vi "GPS -Utility Show Locations.vi"() -> ()   [LabVIEW 2019]
uses:
  <vilib>/Utility/miscctls.llb/LVPoint32TypeDef.ctl
  SUBVIS/ctlGPSColIdxs.ctl
  SUBVIS/InputsGPSTool.ctl
  SUBVIS/ctlMode4GPSTool.ctl
  SUBVIS/ctlSeqFNs -GPSLocation.ctl
  SUBVIS/ctlGPSChangeMrksInputs.ctl
  SUBVIS/ctlInput4PtsColl.ctl
  System.Drawing
  SUBVIS/ctlAddrToGPSInputs.ctl
  C:/Users/WeGo/Documents/GitHub/ERP42mini-v2/GPS/gmap.net/GMAP.NET 8.6/data/GMap.NET.Core.dll
  data/GMap.NET.Core.dll
  SUBVIS/GLBL -GPSLocation.vi
  SUBVIS/GLOBAL -Project MAIN.vi
  C:/Users/WeGo/Documents/GitHub/ERP42mini-v2/GPS/gmap.net/GMAP.NET 8.6/data/GMap.NET.WindowsForms.dll
  data/GMap.NET.WindowsForms.dll
panel:
  in  "Inputs":T1={"ctlMode4GPSTool"=enum."Audit", "Addr"="Talisman Center", "City"="Calgary", "Prov"="Alberta", "Idx"=0, "Lat"="", "Lng"="", "Audited"=FALSE}
  in  "cmbProviders":string(combo)="27" caption="Map Providers"
  in  "tbCtl":enum32{"Audit"}(tab)
  in  "btnCancel":bool
  in  "btnUseMarkerShown":bool
  in  "Refersh":bool
  in  "ClearMarkers":bool
  in  "tbCtlGUI":enum32{"Position", "Pin Drop", "Addr", "Setup"}(tab)
  out "MouseLatDblClck":dbl caption="Lat" format="%#.7f"
  out "MouseLngDblClck":dbl caption="Lng" format="%#.7f"
  out "MouseLat":dbl caption="Lat" format="%#.7f"
  out "MouseLng":dbl caption="Lng" format="%#.7f"
  in  "GetNearPtsDyn":bool
  in  "# Pts":i32=5
  in  "GetNearPts":bool
  in  "PinDropMrkr":T3(ring) caption="Pin Drop Marker"
  out "PinDropLngDblClck":dbl caption="Lng:" format="%#.7f"
  out "PinDropLatDblClck":dbl caption="Lat:" format="%#.7f"
  out "AddrLng":dbl format="%#.7f"
  out "AddrLat":dbl format="%#.7f"
  in  "Get Lat+Lng":bool
  in  "City":string
  in  "Prov":string
  in  "Addr":string="20 Citadel Hills Green NW" caption="Address (Street level)"
  out "InitLoc":string="Calgary, Alberta" caption="Location Start KeyWords"
  out "InitProviders":string="GoogleMap" caption="Starting Provider"
  in  "Mode":T4(ring)
  in  "btnZoom+Center":bool
  in  "SaveImage":bool
  out "ImgPath":string caption="Path"
  in  "Zoom":dbl(slide) scale=0.0..20.0
  in  "tbctlHide":enum32{"Page 1", "Page 2"}(tab)
  out "error out":errorcluster
  in  "error in (no error)":errorcluster
  out "Coords":T5
  in  "EnumMarkerTypes":T3(ring)
  in  "ColIdxs":T6
  in  "Postion":T7
  in  "dotNetGMap":refnum<k24>(container)
  # "ABOVE is Marker LAT, LNG for ADRESS SHOWN:\n\n- If Marker Position is NOT Accurate:\n\n                           (1) 'Clear' the shown marker by clicking on <Clear Markers>\n\n                           (2) 'Double-Click' on Map to drop a Pin at New Position\n\n- If Marker Position is Accurate:\n                           \n                              Click Use the 'Marker Position' Shown to accept you new position"
  # "DYNAMIC"
  # "Mouse <Move> Coordinates"
  # "STATIC"
  # "Mouse <Dbl Clck> Coordinates"
  # "STEP 1. Dbl Clck Position"
  # "STEP 2. Edit Marker"
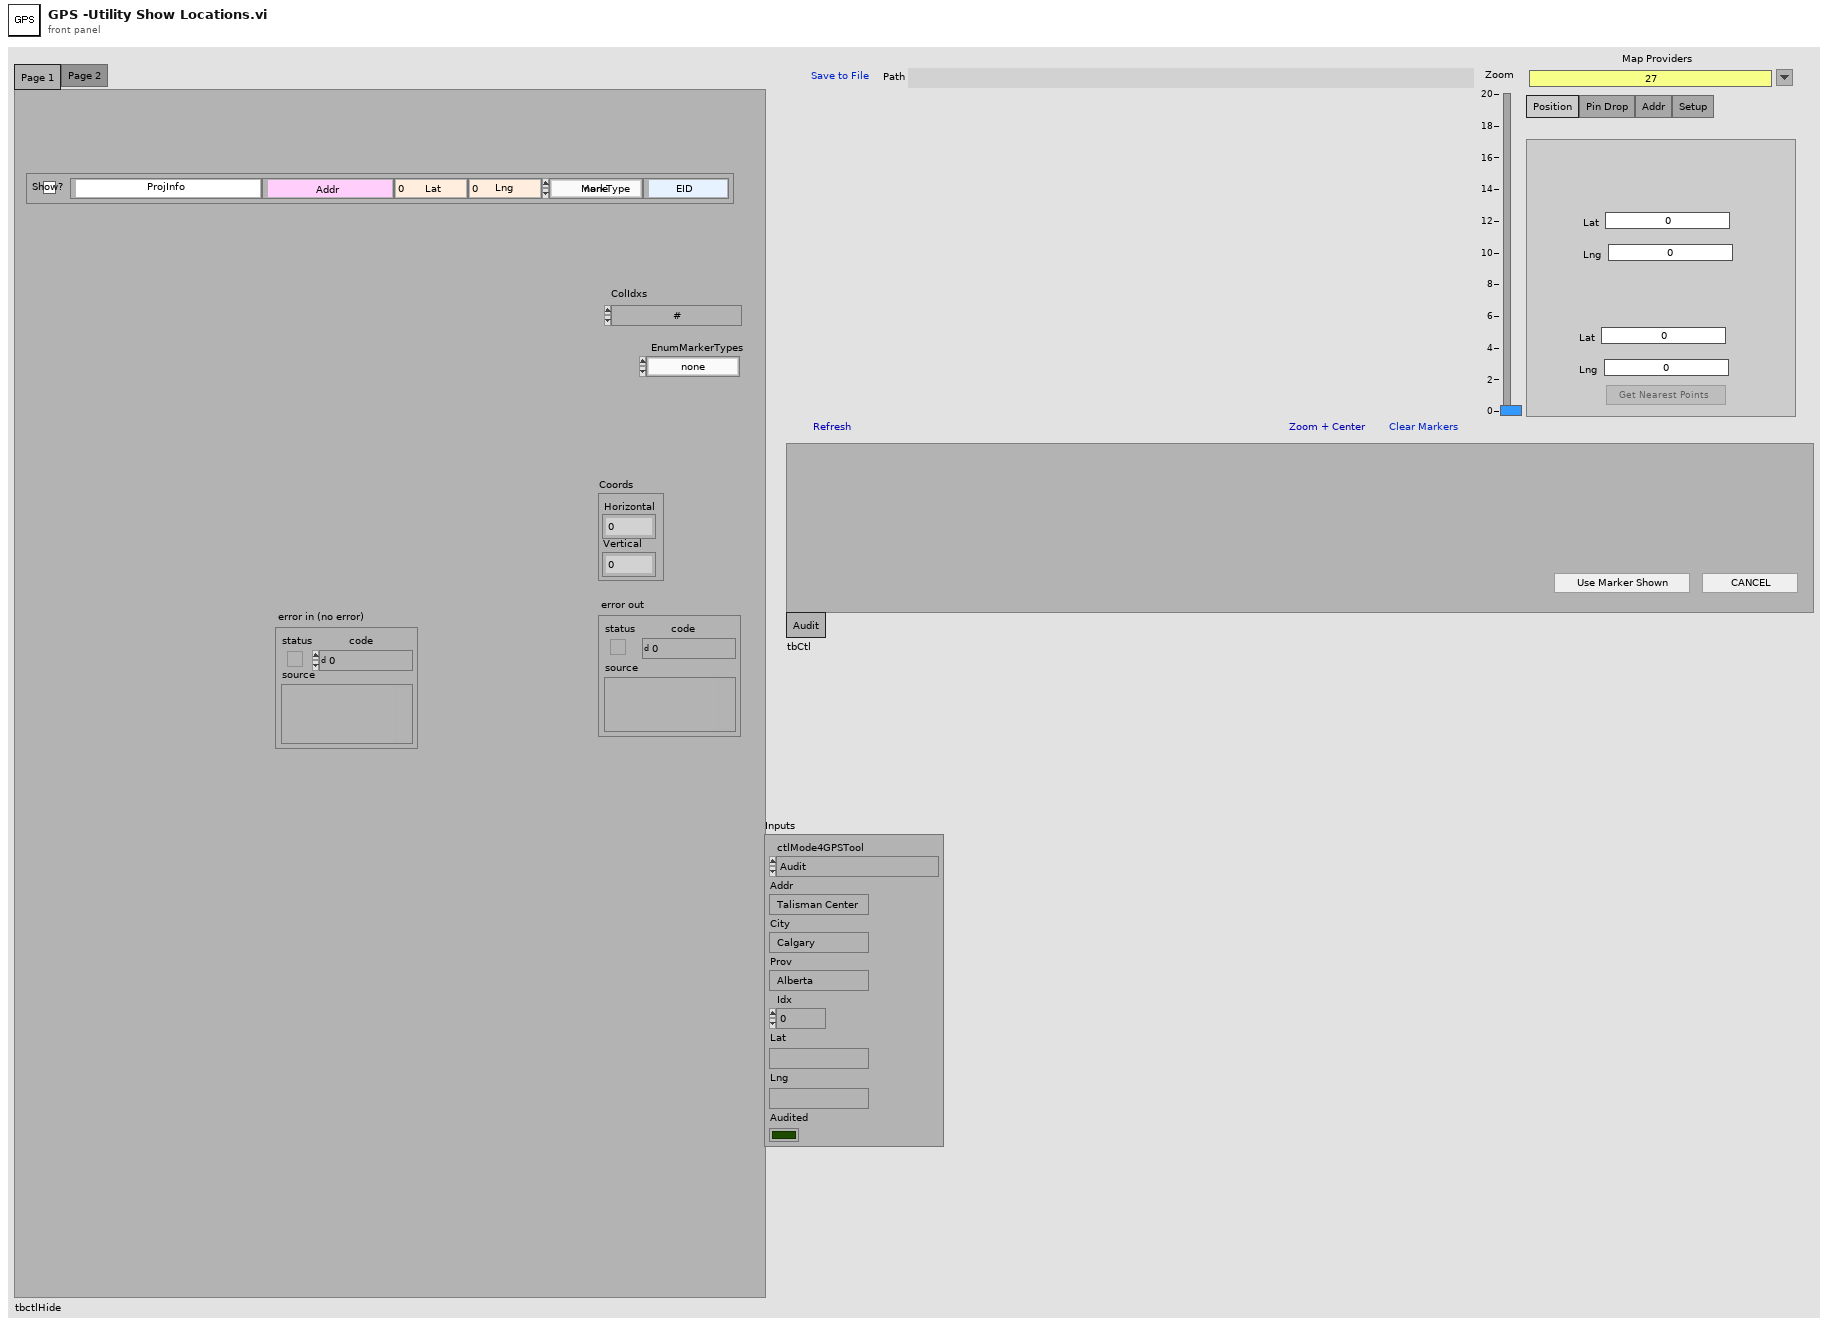
[diagram p1: front panel]
types:
  T1 = typedef "InputsGPSTool.ctl" = cluster{"ctlMode4GPSTool":T2, "Addr":string, "City":string, "Prov":string, "Idx":i32, "Lat":string, "Lng":string, "Audited":bool}
  T2 = typedef "ctlMode4GPSTool.ctl" = enum16{"NA", "Audit"}
  T3 = enum16{"none", "arrow", "blue", "blue_small", "blue_dot", "blue_pushpin", "brown_small", "gray_small", "green", "green_small", "green_dot", "green_pushpin", "green_big_go", "yellow", "yellow_small", "yellow_dot", "yellow_big_pause", "yellow_pushpin", "lightblue", "lightblue_dot", "lightblue_pushpin", "orange", "orange_small", "orange_dot", "pink", "pink_dot", "pink_pushpin", "purple", "purple_small", "purple_dot", "purple_pushpin", "red", "red_small", "red_dot", "red_pushpin", "red_big_stop", "black_small", "white_small"}
  T4 = enum16{"ServerOnly", "ServerAndCache", "CacheOnly"}
  T5 = typedef "LVPoint32TypeDef.ctl" = cluster{"Horizontal":i32, "Vertical":i32}
  T6 = typedef "ctlGPSColIdxs.ctl" = enum16{"#", "Vw", "Year", "Project Info", "Address", "Lat", "Lng", "Icon -Maps", "Icon -Custom", "EIDProj", "EIDAddr", "OnMap"}
  T7 = cluster{"Show?":bool, "ProjInfo":string, "Addr":string, "Lat":dbl, "Lng":dbl, "MarkType":enum16{"none", "arrow", "blue", "blue_small", "blue_dot", "blue_pushpin", "brown_small", "gray_small", "green", "green_small", "green_dot", "green_pushpin", "green_big_go", "yellow", "yellow_small", "yellow_dot", "yellow_big_pause", "yellow_pushpin", "lightblue", "lightblue_dot", "lightblue_pushpin", "orange", "orange_small", "orange_dot", "pink", "pink_dot", "pink_pushpin", "purple", "purple_small", "purple_dot", "purple_pushpin", "red", "red_small", "red_dot", "red_pushpin", "red_big_stop", "black_small", "white_small"}, "EID":string}
  T8 = typedef "ctlSeqFNs -GPSLocation.ctl" = enum16{"pre-init", "preinit01", "preinit02", "preinit03", "preinit04", "preinit05", "init", "idle", "GUI -Pop Menu", "GUI -Add Marker Combo", "GUI -Annotate Grid", "ALIGN COLS", "SET -Provider", "SET -SCALE", "OVERLAY -ADD", "POINTS -CREATE LIST (Container)", "MARKERS -CREATE LIST", "MAP -MARKER Add Or Rmv", "DOWNLOAD -Project Addr", "MAP -Marker Update", "MAP -Save", "MAP -Markers Autofit", "MAP -Addr to Lat + Lng", "MAP -Markers Clear", "PIN DROP -Get Nearest", "AUDIT -Use Marker Shown", "error", "exit"}
  T9 = cluster{"Idx|Addr|City|Prov|Lng|Lat|Checked":string[], "tbCtlGUI":refnum<vi>, "PinDropLatDblClck":refnum<vi>, "PinDropLngDblClck":refnum<vi>, "Cols4Show":i32, "ColHdrs":string[], "ColNos":i32[], "ColWidths":i32[], "AligmntEnum":i32[], "MouseLat":refnum<vi>, "MouseLng":refnum<vi>, "RefScale":refnum<vi>, "RefcmbProviders":refnum<vi>, "RefMode":refnum<vi>, "RefInitProvider":refnum<vi>, "EvntRefGMap":refnum<k27>, "arrRefProviders":refnum<k24>[], "arrProviderNms":string[], "RefInitLoc":refnum<vi>, "dotNetGMap":refnum<k24>, "PathCurr":path, "VIRef":refnum<vi>, "arrOverlayNames":string[], "arrOverlayRefs":refnum<k24>[], "RefPointsColl":refnum<k24>, "arrLatLngActv":dbl[][], "arrPointKeyWordOrID":string[], "EvntRefVsData":refnum<k27>, "MouseLatDblClck":refnum<vi>, "MouseLngDblClck":refnum<vi>, "Inputs":T1}
  T10 = enum8{"Enabled", "Disabled", "Disabled and Grayed Out"}
  T11 = typedef "ctlInput4PtsColl.ctl" = cluster{"arrLatLngActv":dbl[][], "ptKeyorID":string[], "Add":bool}
  T12 = cluster{"arrOverlayRefs":refnum<k24>[], "RefPointsColl in":refnum<k24>, "arrPointKeyWordOrID":string[], "PtLatLn+KywrdOrID":T11, "arrLatLngActv":dbl[][]}
  T13 = typedef "ctlAddrToGPSInputs.ctl" = cluster{"City":string, "State":string, "Addr":string, "EID":string}
  T14 = cluster{" # Pts":i32, "PinDropLatDblClck":dbl, "PinDropLngDblClck":dbl, "AddrLat":dbl, "AddrLng":dbl, "tbVw":enum32{"Position", "Pin Drop", "Addr", "Setup"}}
  T15 = cluster{refnum<vi>[], "tbCtlGUI":refnum<vi>, "queue out":refnum<queue>}
  T16 = typedef "ctlGPSChangeMrksInputs.ctl" = cluster{"r|c":i32[], "ID":string, "MrkName":string}
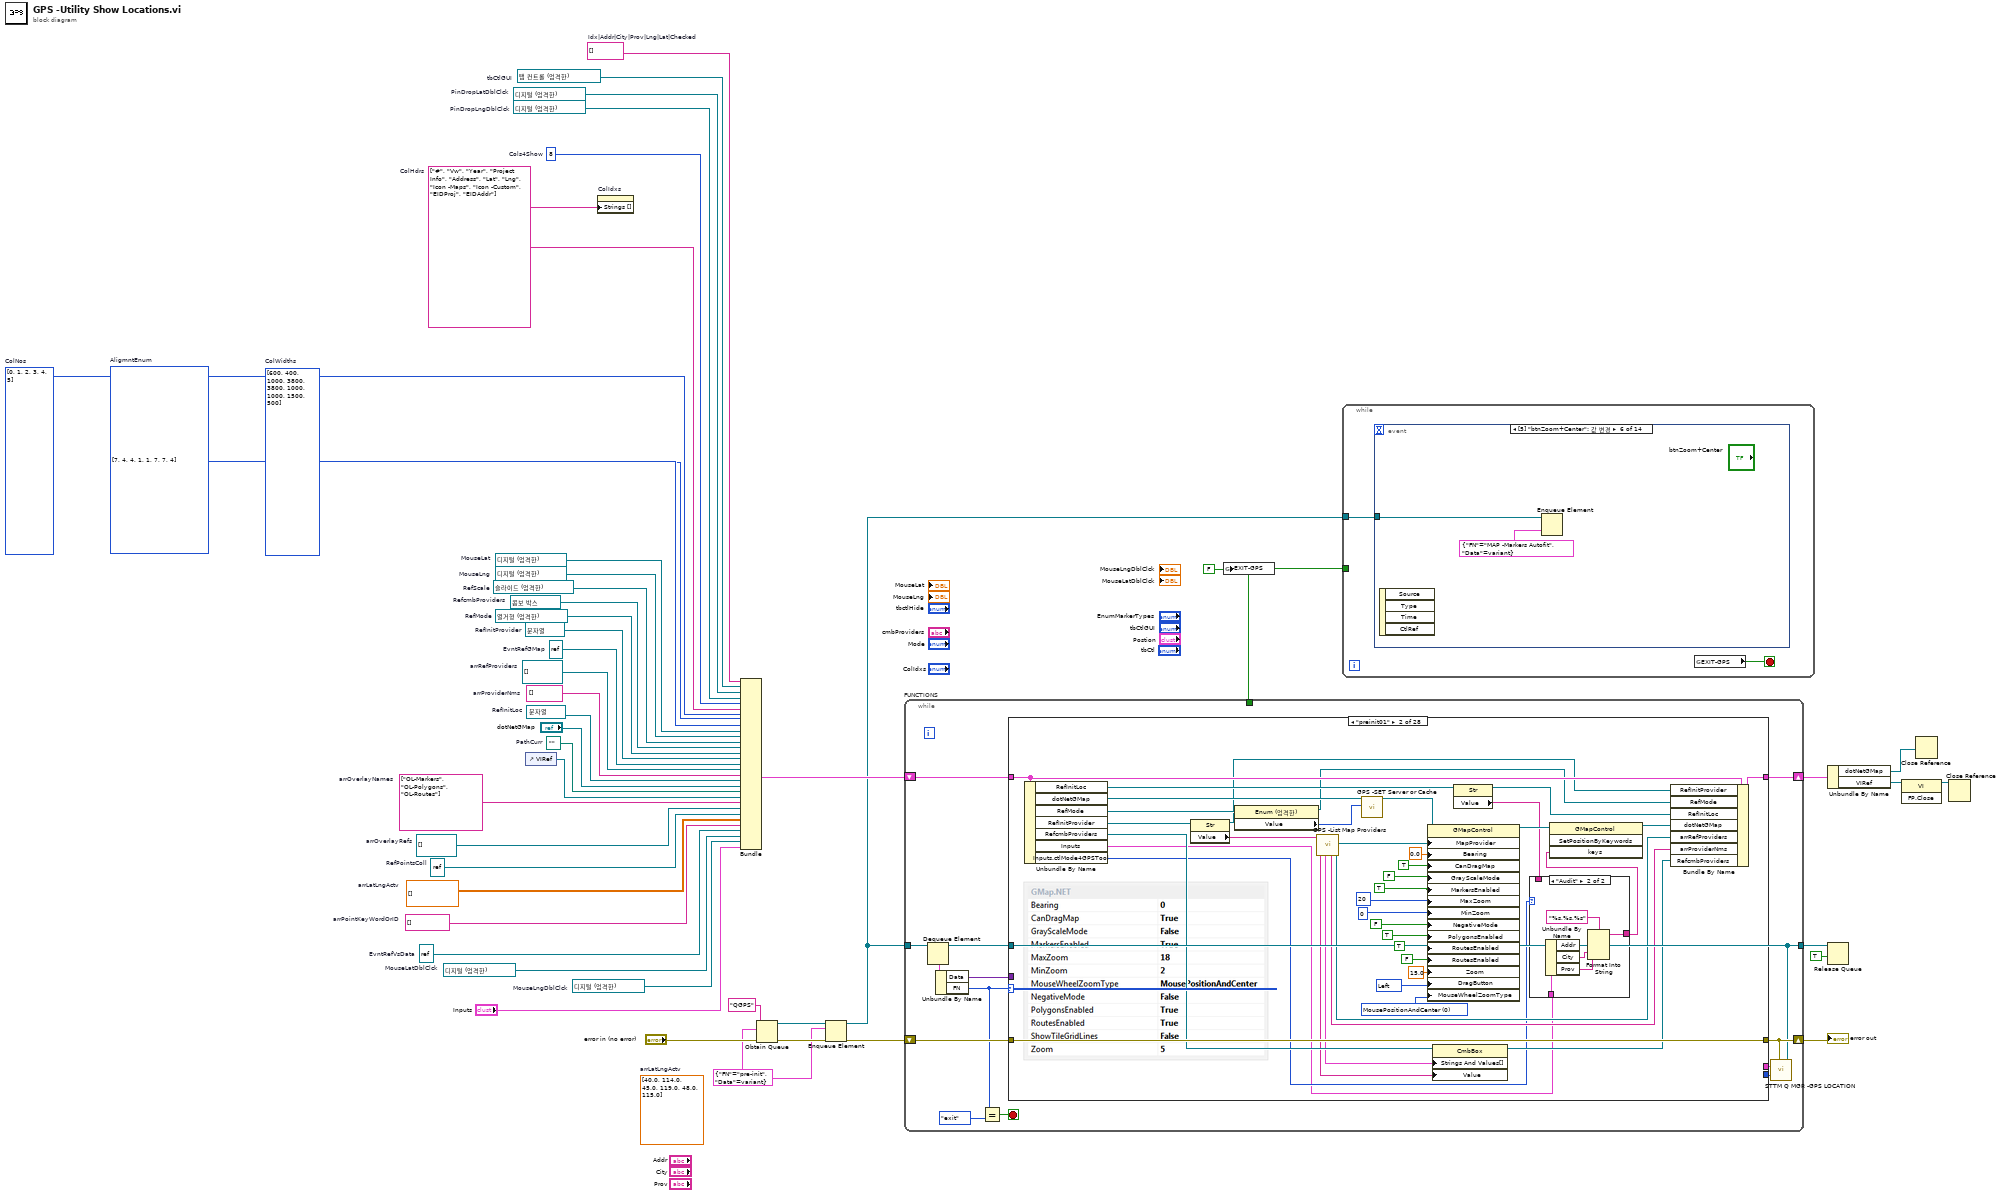
[diagram p0: block diagram]
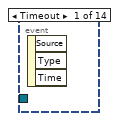
[diagram p2: hidden frame]
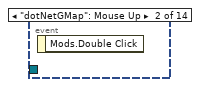
[diagram p3: hidden frame]
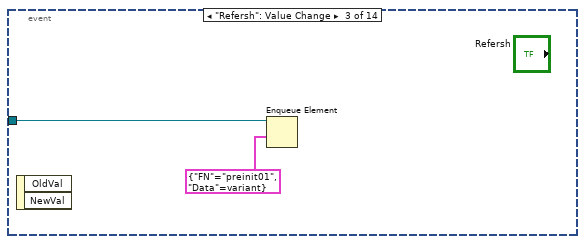
[diagram p4: hidden frame]
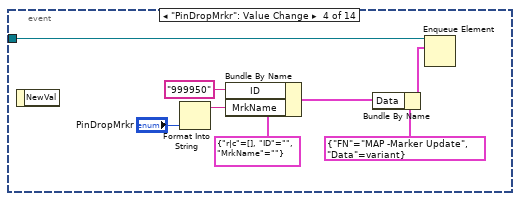
[diagram p5: hidden frame]
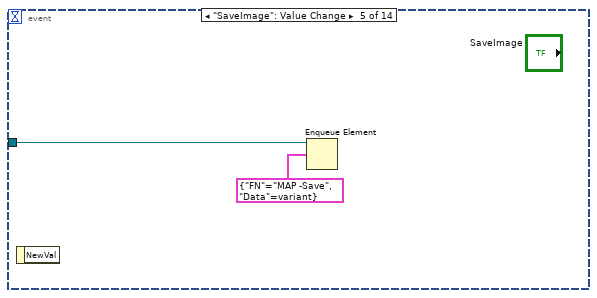
[diagram p6: hidden frame]
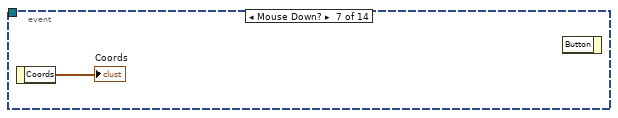
[diagram p7: hidden frame]
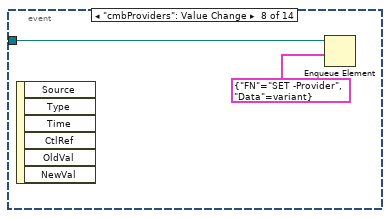
[diagram p8: hidden frame]
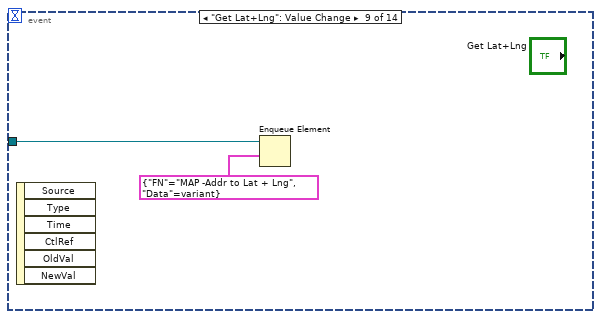
[diagram p9: hidden frame]
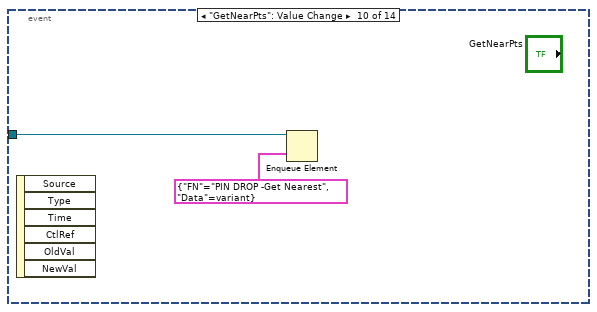
[diagram p10: hidden frame]
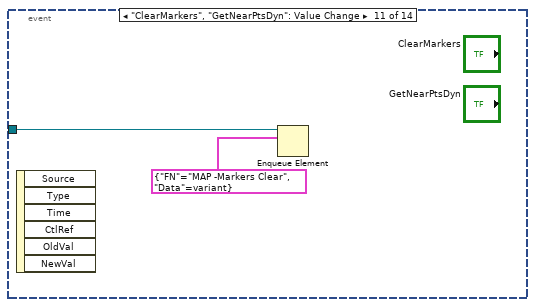
[diagram p11: hidden frame]
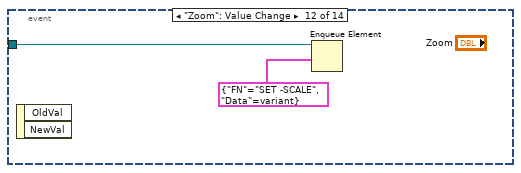
[diagram p12: hidden frame]
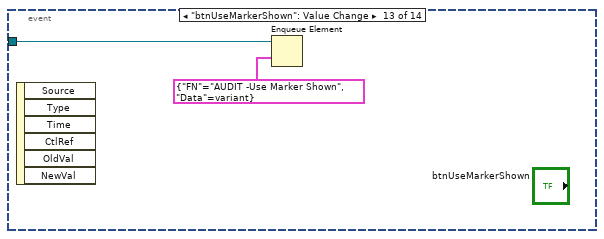
[diagram p13: hidden frame]
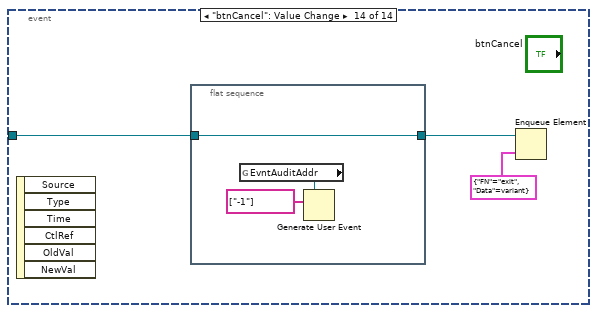
[diagram p14: hidden frame]
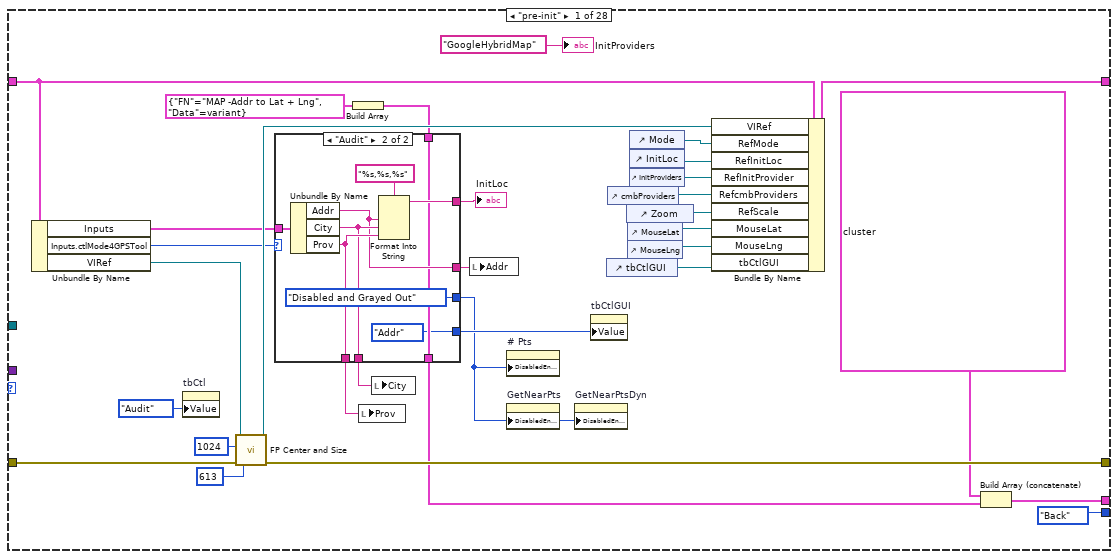
[diagram p15: hidden frame]
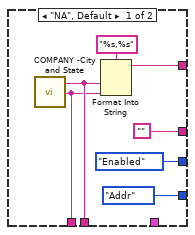
[diagram p16: hidden frame]
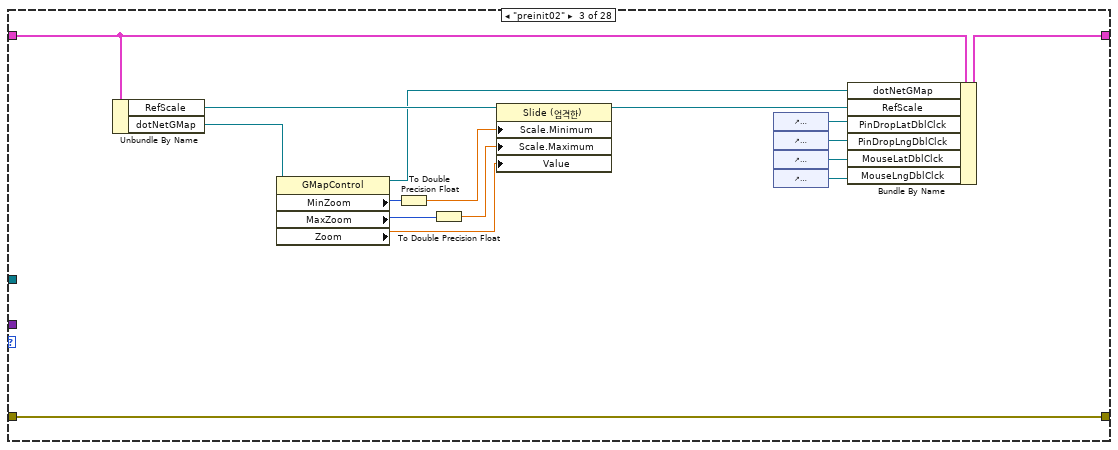
[diagram p18: hidden frame]
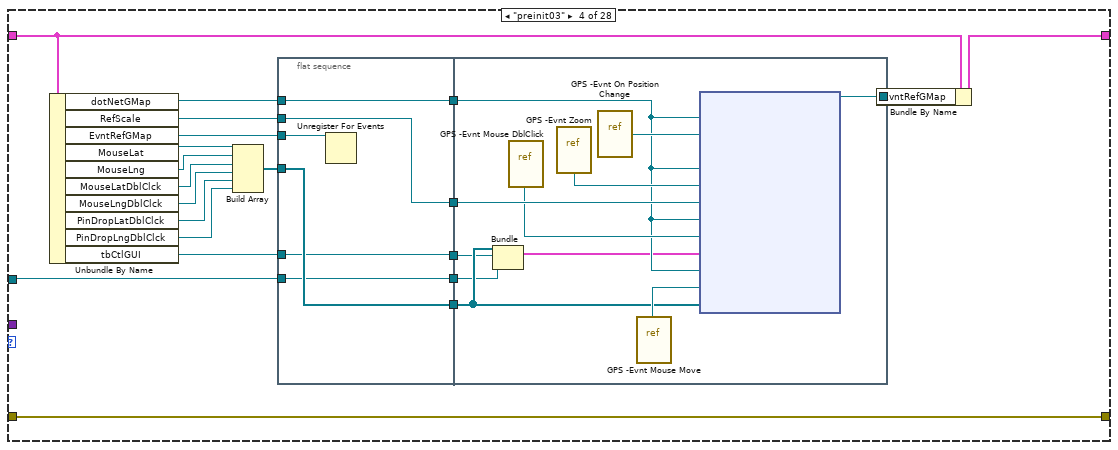
[diagram p19: hidden frame]
diagram:
  w2 = string[] []  # Idx|Addr|City|Prov|Lng|Lat|Checked
  w4 = refnum<vi> refnum  # tbCtlGUI
  w6 = refnum<vi> refnum  # PinDropLngDblClck
  w5 = refnum<vi> refnum  # PinDropLatDblClck
  w8 = refnum<vi> refnum  # MouseLngDblClck
  w9 = refnum<vi> refnum  # MouseLatDblClck
  w10 = refnum<k27> refnum  # EvntRefVsData
  w11 = 8  # Cols4Show
  w7 = string[] ["#", "Vw", "Year", "Project Info", "Address", "Lat", "Lng", "Icon -Maps", "Icon -Custom", "EIDProj", "EIDAddr"]  # ColHdrs
  w14 = i32[] [7, 4, 4, 1, 1, 7, 7, 4] items=["flexAlignLeftTop", "flexAlignLeftCenter", "flexAlignLeftBottom", "flexAlignCenterTop", "flexAlignCenterCenter", "flexAlignCenterBottom", "flexAlignRightTop", "flexAlignRightCenter", "flexAlignRightBottom", "flexAlignGeneral", "flexAlignGeneralTop", "flexAlignGeneralCenter", "flexAlignGeneralBottom"]  # AligmntEnum
  w12 = i32[] [0, 1, 2, 3, 4, 5]  # ColNos
  w13 = i32[] [600, 400, 1000, 3800, 3800, 1000, 1000, 1500, 500]  # ColWidths
  w15 = string[] []  # arrPointKeyWordOrID
  (unwired) dbl[][] [[40.0, 114.0], [45.0, 119.0], [48.0, 115.0]]  # arrLatLngActv
  w16 = dbl[][] []  # arrLatLngActv
  w17 = refnum<k24> refnum  # RefPointsColl
  w18 = refnum<k24>[] []  # arrOverlayRefs
  w19 = string[] ["OL-Markers", "OL-Polygons", "OL-Routes"]  # arrOverlayNames
  w20 = refnum<vi> refnum  # MouseLat
  w21 = refnum<vi> refnum  # MouseLng
  w22 = refnum<vi> refnum  # RefScale
  w27 = refnum<vi> refnum  # RefcmbProviders
  w25 = refnum<vi> refnum  # RefInitProvider
  w26 = refnum<vi> refnum  # RefMode
  w24 = refnum<vi> refnum  # RefInitLoc
  w28 = refnum<k27> refnum  # EvntRefGMap
  w30 = string[] []  # arrProviderNms
  w29 = refnum<k24>[] []  # arrRefProviders
  w32 = cluster{"FN":T8, "Data":variant} {"FN"=enum."pre-init", "Data"=variant} ("element")
  w40 = FALSE ("EXIT-GPS")
  w42 = path ""  # PathCurr
  n1 = control-ref of="VIRef"() -> (w37:refnum<vi>)
  n2 = property on="ColIdxs" class="Enum (strict)"("Strings []"=w7) -> ()  [unwired: 2 in, 2 out]
  n3 = Bundle("Idx|Addr|City|Prov|Lng|Lat|Checked"=w2, "tbCtlGUI"=w4, "PinDropLatDblClck"=w5, "PinDropLngDblClck"=w6, "Cols4Show"=w11, "ColHdrs"=w7, "ColNos"=w12, "ColWidths"=w13, "AligmntEnum"=w14, "MouseLat"=w20, "MouseLng"=w21, "RefScale"=w22, "RefcmbProviders"=w27, "RefMode"=w26, "RefInitProvider"=w25, "EvntRefGMap"=w28, "arrRefProviders"=w29, "arrProviderNms"=w30, "RefInitLoc"=w24, "dotNetGMap"="dotNetGMap", "PathCurr"=w42, "VIRef"=w37, "arrOverlayNames"=w19, "arrOverlayRefs"=w18, "RefPointsColl"=w17, "arrLatLngActv"=w16, "arrPointKeyWordOrID"=w15, "EvntRefVsData"=w10, "MouseLatDblClck"=w9, "MouseLngDblClck"=w8, "Inputs"="Inputs") -> (w44:T9)  [unwired: 1 in]
  n4 = Obtain Queue(name (unnamed)="QGPS", element data type=w32) -> (queue out=w34:refnum<queue>)  [unwired: 3 in, 2 out]
  n5 = Enqueue Element(queue=w34, element=w32) -> (queue out=w23:refnum<queue>)  [unwired: 2 in, 2 out]
  n6 = while "FUNCTIONS" {
    shift-right: [w55] -> w41
    shift-left: "error in (no error)" -> [w58]
    shift-right: [w56] -> w39
    shift-left: w44 -> [w57]
    tunnel: w40 -> [_]
    tunnel: w23 -> [w54]
    tunnel: [w46] -> w31
    stop <- w51 stop-if-true
    n7 = Dequeue Element(queue=w54) -> (queue out=w46:refnum<queue>, element=w53:cluster{"FN":T8, "Data":variant})  [unwired: 2 in, 2 out]
    n8 = Unbundle By Name(w53) -> ("Data"=w52:variant, "FN"=w50:T8)
    n9 = Equal?(x=w50, y=ctlSeqFNs_-GPSLocation."exit") -> (x = y?=w51:bool)
    n10 = case shown="\"preinit01\"" w50 {
      tunnel: w58 -> [w89 w145 w168 w189 w208 w209 w212 w215 w216 w219 w221 w223 w235 w243 w251 w262 w264 w281 w283 w297 w308 w317 w350 w360 w361 w424 w426 w429]
      tunnel: [w88 w145 w168 w189 w208 w209 w212 w215 w216 w219 w221 w223 w235 w243 w251 w262 w264 w281 w283 w297 w308 w317 w350 w360 w361 w423 w426 w429] -> w55
      tunnel: w57 -> [w84 w144 w160 w187 w207 w210 w211 w214 w217 w218 w220 w222 w232 w240 w249 w259 w263 w278 w282 w288 w300 w316 w329 w356 w371 w414 w425 w428]
      tunnel: [w82 w142 w157 w186 w207 w210 w211 w214 w217 w218 w220 w222 w231 w238 w247 w261 w263 w276 w282 w287 w299 w316 w329 w355 w370 w414 w425 w428] -> w56
      tunnel: w52 -> [_ _ _ _ _ _ _ _ _ _ _ _ _ _ _ _ _ w280 _ _ _ _ _ _ _ _ _ _]
      tunnel: [w62 _ _ _ _ _ _ _ _ _ _ _ _ _ _ _ _ w274 _ _ _ _ w334 _ w369 _ _ _] -> w48
      tunnel: [enum16{"Back", "Front", "Replace"}."Back" ("Enum") _ _ _ _ _ _ _ _ _ _ _ _ _ _ _ _ _ _ _ _ _ _ _ _ _ _ _] -> w47
      tunnel: w46 -> [_ _ _ w169 _ _ _ _ _ _ _ _ _ _ _ _ _ _ _ _ _ _ _ _ _ _ _ _]
      frame "pre-init" {
        n11 = Unbundle By Name(w84) -> ("Inputs"=w71:T1, "Inputs.ctlMode4GPSTool"=w72:T2, "VIRef"=w87:refnum<vi>)
        n12 = property on="tbCtl" class="TabCtl (strict)"("Value"=enum32{"Audit", "Page 1"}."Audit" ("tbCtl")) -> ()  [unwired: 2 in, 2 out]
        n13 = call "FP Center and Size.vi"("error in (no error)"=w89, "bottom"=i16 613, "right"=i16 1024, "VIRefNum  IN"=w87) -> ("error out"=w88:errorcluster, "VIRefNum OUT"=w83:refnum<vi>)  [unwired: 6 in]
        n14 = Build Array(cluster{"FN":T8, "Data":variant} {"FN"=enum."MAP -Addr to Lat + Lng", "Data"=variant} ("element")) -> (w65:cluster{"FN":T8, "Data":variant}[])
        n15 = case shown="\"Audit\"" w72 {
          tunnel: w71 -> [_ w106]
          tunnel: [w94 w105] -> w70
          tunnel: [w96 w102] -> w69
          tunnel: [w95 w103] -> w68
          tunnel: ["" w101] -> w67
          tunnel: w65 -> [_ w100]
          tunnel: [_ w100] -> w63
          tunnel: [enum32{"Position", "Pin Drop", "Addr", "Setup"}."Addr" ("tbCtlGUI") enum32{"Position", "Pin Drop", "Addr", "Setup"}."Addr" ("tbCtlGUI")] -> w60
          tunnel: [T10."Enabled" ("Disabled") T10."Disabled and Grayed Out" ("Disabled")] -> w59
          frame "NA", Default {
            n16 = call "COMPANY -City and State.vi"() -> ("Prov|State"=w95:string, "City"=w96:string)  [unwired: 10 in]
            n17 = Format Into String(format string="%s,%s", w96, w95) -> (resulting string=w94:string)  [unwired: 2 in, 1 out]
          }
          frame "Audit" {
            n18 = Unbundle By Name(w106) -> ("Addr"=w101:string, "City"=w102:string, "Prov"=w103:string)
            n19 = Format Into String(format string="%s,%s,%s", w101, w102, w103) -> (resulting string=w105:string)  [unwired: 2 in, 1 out]
          }
        }
        "InitLoc" <- w70
        n20 = local write "Prov"(w68) -> ()
        n21 = local write "City"(w69) -> ()
        n22 = local write "Addr"(w67) -> ()
        n23 = property on="# Pts" class="DigNum (strict)"("DisabledEnum"=w59) -> ()  [unwired: 2 in, 2 out]
        n24 = property on="GetNearPts" class="Bool"("DisabledEnum"=w59) -> ()  [unwired: 2 in, 2 out]
        n25 = property on="GetNearPtsDyn" class="Bool"("DisabledEnum"=w59) -> ()  [unwired: 2 in, 2 out]
        n26 = property on="tbCtlGUI" class="TabCtl (strict)"("Value"=w60) -> ()  [unwired: 2 in, 2 out]
        n27 = control-ref of="tbCtlGUI"() -> (w73:refnum<vi>)
        n28 = control-ref of="cmbProviders"() -> (w78:refnum<vi>)
        n29 = control-ref of="Zoom"() -> (w77:refnum<vi>)
        n30 = control-ref of="MouseLat"() -> (w76:refnum<vi>)
        n31 = control-ref of="MouseLng"() -> (w75:refnum<vi>)
        n32 = control-ref of="Mode"() -> (w81:refnum<vi>)
        n33 = control-ref of="InitLoc"() -> (w80:refnum<vi>)
        n34 = control-ref of="InitProviders"() -> (w79:refnum<vi>)
        n35 = Bundle By Name(cluster=w84, "VIRef"=w83, "RefMode"=w81, "RefInitLoc"=w80, "RefInitProvider"=w79, "RefcmbProviders"=w78, "RefScale"=w77, "MouseLat"=w76, "MouseLng"=w75, "tbCtlGUI"=w73) -> (w82:T9)
        n36 = Build Array (concatenate)(cluster{"FN":T8, "Data":variant}[] [{"FN"=enum."preinit01", "Data"=variant}, {"FN"=enum."preinit02", "Data"=variant}, {"FN"=enum."preinit03", "Data"=variant}, {"FN"=enum."preinit04", "Data"=variant}, {"FN"=enum."preinit05", "Data"=variant}, {"FN"=enum."init", "Data"=variant}, {"FN"=enum."idle", "Data"=variant}, {"FN"=enum."OVERLAY -ADD", "Data"=variant}, {"FN"=enum."POINTS -CREATE LIST (Container)", "Data"=variant}, {"FN"=enum."DOWNLOAD -Project Addr", "Data"=variant}] ("QFNs"), w63) -> (w62:cluster{"FN":T8, "Data":variant}[])
        "InitProviders" <- "GoogleHybridMap" ("InitProviders")
      }
      frame "preinit01" {
        w114 = 1048576 items=["None"=0, "Left"=1048576, "Right"=2097152, "Middle"=4194304, "XButton1"=8388608, "XButton2"=16777216] ("DragButton")
        w131 = 0 items=["MousePositionAndCenter", "MousePositionWithoutCenter", "ViewCenter"] ("MouseWheelZoomType")
        n37 = Unbundle By Name(w144) -> ("RefInitLoc"=w141:refnum<vi>, "dotNetGMap"=w133:refnum<k24>, "RefMode"=w123:refnum<vi>, "RefInitProvider"=w121:refnum<vi>, "RefcmbProviders"=w119:refnum<vi>, "Inputs"=w109:T1, "Inputs.ctlMode4GPSTool"=w110:T2)
        n38 = property class="Str"(reference=w121) -> (reference out=w116:refnum<vi>, "Value"=w120:string)  [unwired: 1 in, 1 out]
        n39 = property class="Enum (엄격한)"(reference=w123) -> (reference out=w115:refnum<vi>, "Value"=w122:T4)  [unwired: 1 in, 1 out]
        n40 = call "GPS -List Map Providers.vi"("InitProviders"=w120) -> ("IdxInitPrvd"=w113:string, "SelProvider"=w111:refnum<k24>, "cmbProviders"=w118:cluster{"Name":string, string}[], "arrRefProviders"=w139:refnum<k24>[], "arr1DProviders"=w140:string[])  [unwired: 6 in]
        n41 = call "GPS -SET Server or Cache.vi"("Mode"=w122, ".NET Refnum in"=w133) -> (".NET Refnum out"=w132:refnum<k24>)  [unwired: 9 in]
        n42 = property class="GMapControl"(reference=w132, "MapProvider"=w111, "Bearing"=sgl 0.0, "CanDragMap"=TRUE, "GrayScaleMode"=FALSE ("CanDragMap"), "MarkersEnabled"=TRUE, "MaxZoom"=20, "MinZoom"=0, "NegativeMode"=FALSE, "PolygonsEnabled"=TRUE, "RoutesEnabled"=TRUE, "RoutesEnabled"=FALSE, "Zoom"=15.0, "DragButton"=w114, "MouseWheelZoomType"=w131) -> (reference out=w112:refnum<k24>)  [unwired: 1 in, 1 out]
        n43 = property class="CmbBox"(reference=w119, "Strings And Values[]"=w118, "Value"=w113) -> (reference out=w117:refnum<vi>)  [unwired: 1 in, 1 out]
        n44 = property class="Str"(reference=w141) -> (reference out=w124:refnum<vi>, "Value"=w107:string)  [unwired: 1 in, 1 out]
        n45 = case shown="\"Audit\"" w110 {
          tunnel: w109 -> [_ w151]
          tunnel: [w146 w147] -> w108
          tunnel: w107 -> [w146 _]
          frame "NA", Default {
          }
          frame "Audit" {
            n46 = Unbundle By Name(w151) -> ("Addr"=w152:string, "City"=w150:string, "Prov"=w149:string)
            n47 = Format Into String(format string="%s,%s,%s", w152, w150, w149) -> (resulting string=w147:string)  [unwired: 2 in, 1 out]
          }
        }
        n48 = invoke class="GMapControl" method="SetPositionByKeywords"(reference=w112, "keys"=w108) -> (reference out=w143:refnum<k24>)  [unwired: 2 in, 3 out]
        n49 = Bundle By Name(cluster=w144, "RefInitProvider"=w116, "RefMode"=w115, "RefInitLoc"=w124, "dotNetGMap"=w143, "arrRefProviders"=w139, "arrProviderNms"=w140, "RefcmbProviders"=w117) -> (w142:T9)
      }
      frame "preinit02" {
        n50 = Unbundle By Name(w160) -> ("RefScale"=w166:refnum<vi>, "dotNetGMap"=w167:refnum<k24>)
        n51 = property class="GMapControl"(reference=w167) -> (reference out=w158:refnum<k24>, "MinZoom"=w164:i32, "MaxZoom"=w163:i32, "Zoom"=w165:dbl)  [unwired: 1 in, 1 out]
        n52 = To Double Precision Float(number=w164) -> (double precision float=w162:dbl)
        n53 = To Double Precision Float(number=w163) -> (double precision float=w161:dbl)
        n54 = property class="Slide (엄격한)"(reference=w166, "Scale.Minimum"=w162, "Scale.Maximum"=w161, "Value"=w165) -> (reference out=w159:refnum<vi>)  [unwired: 1 in, 1 out]
        n55 = control-ref of="PinDropLatDblClck"() -> (w156:refnum<vi>)
        n56 = control-ref of="PinDropLngDblClck"() -> (w155:refnum<vi>)
        n57 = control-ref of="MouseLatDblClck"() -> (w154:refnum<vi>)
        n58 = control-ref of="MouseLngDblClck"() -> (w153:refnum<vi>)
        n59 = Bundle By Name(cluster=w160, "dotNetGMap"=w158, "RefScale"=w159, "PinDropLatDblClck"=w156, "PinDropLngDblClck"=w155, "MouseLatDblClck"=w154, "MouseLngDblClck"=w153) -> (w157:T9)
      }
      frame "preinit03" {
        n60 = Unbundle By Name(w187) -> ("dotNetGMap"=w188:refnum<k24>, "RefScale"=w182:refnum<vi>, "EvntRefGMap"=w181:refnum<k27>, "MouseLat"=w180:refnum<vi>, "MouseLng"=w179:refnum<vi>, "MouseLatDblClck"=w176:refnum<vi>, "MouseLngDblClck"=w175:refnum<vi>, "PinDropLatDblClck"=w174:refnum<vi>, "PinDropLngDblClck"=w173:refnum<vi>, "tbCtlGUI"=w171:refnum<vi>)
        n61 = Build Array(w180, w179, w176, w175, w174, w173) -> (w177:refnum<vi>[])
        n62 = flat-sequence {
          tunnel: w188 -> [w195]
          tunnel: [w195] -> w184
          tunnel: [w194] -> w183
          tunnel: w182 -> [w194]
          tunnel: w181 -> [w193]
          tunnel: [w192] -> w178
          tunnel: w177 -> [w192]
          tunnel: [w191] -> w172
          tunnel: w171 -> [w191]
          tunnel: [w190] -> w170
          tunnel: w169 -> [w190]
          tunnel: [w206] -> w185
          tunnel: w184 -> [w201]
          tunnel: w183 -> [w203]
          tunnel: w178 -> [w199]
          tunnel: w172 -> [w198]
          tunnel: w170 -> [w196]
          frame #0 {
            n63 = Unregister For Events(event registration refnum=w193) -> ()  [unwired: 1 in, 1 out]
          }
          frame #1 {
            n64 = Bundle(w199, "tbCtlGUI"=w198, "queue out"=w196) -> (w197:T15)  [unwired: 1 in]
            n65 = vi-ref "GPS -Evnt Mouse DblClick.vi"() -> ("vi reference"=w202:refnum<vi>)
            n66 = vi-ref "GPS -Evnt Zoom.vi"() -> ("vi reference"=w204:refnum<vi>)
            n67 = vi-ref "GPS -Evnt On Position Change.vi"() -> ("vi reference"=w205:refnum<vi>)
            n68 = vi-ref "GPS -Evnt Mouse Move.vi"() -> ("vi reference"=w200:refnum<vi>)
            n69 = node(w201, w205, w201, w204, w203, w201, w202, w197, w201, w200, w199) -> (w206:refnum<k27>)  [unwired: 3 in, 1 out]
          }
        }
        n70 = Bundle By Name(cluster=w187, "EvntRefGMap"=w185) -> (w186:T9)
      }
      frame "preinit04" {
      }
      frame "preinit05" {
      }
      frame "init" {
      }
      frame "idle" {
        n71 = Wait Until Next ms Multiple(millisecond multiple=u32 100) -> ()  [unwired: 1 out]
      }
      frame "GUI -Pop Menu" {
      }
      frame "GUI -Add Marker Combo" {
      }
      frame "GUI -Annotate Grid" {
      }
      frame "ALIGN COLS" {
      }
      frame "SET -Provider" {
        n72 = Unbundle By Name(w232) -> ("dotNetGMap"=w233:refnum<k24>, "arrRefProviders"=w226:refnum<k24>[], "arrProviderNms"=w229:string[], "RefcmbProviders"=w234:refnum<vi>)
        n73 = property class="CmbBox"(reference=w234) -> (reference out=w227:refnum<vi>, "Text.Text"=w230:string)  [unwired: 1 in, 1 out]
        n74 = Search 1D Array(1D array=w229, element=w230) -> (index of element=w228:i32)  [unwired: 1 in]
        n75 = Index Array(array=w226, index=w228) -> (element=w225:refnum<k24>)
        n76 = property class="GMapControl"(reference=w233, "MapProvider"=w225) -> (reference out=w224:refnum<k24>)  [unwired: 1 in, 1 out]
        n77 = Bundle By Name(cluster=w232, "dotNetGMap"=w224, "arrRefProviders"=w226, "RefcmbProviders"=w227) -> (w231:T9)
      }
      frame "SET -SCALE" {
        n78 = Unbundle By Name(w240) -> ("RefScale"=w241:refnum<vi>, "dotNetGMap"=w242:refnum<k24>)
        n79 = property class="Slide (엄격한)"(reference=w241) -> (reference out=w239:refnum<vi>, "Value"=w236:dbl)  [unwired: 1 in, 1 out]
        n80 = property class="GMapControl"(reference=w242, "Zoom"=w236) -> (reference out=w237:refnum<k24>)  [unwired: 1 in, 1 out]
        n81 = Bundle By Name(cluster=w240, "RefScale"=w239, "dotNetGMap"=w237) -> (w238:T9)
      }
      frame "OVERLAY -ADD" {
        n82 = Unbundle By Name(w249) -> ("dotNetGMap"=w246:refnum<k24>, "arrOverlayNames"=w250:string[])
        n83 = for {
          tunnel: w250 -> [w258] mode=indexing
          tunnel: [w252] -> w248 mode=indexing
          shift-right: [w255] -> w245
          shift-left: w246 -> [w257]
          tunnel: TRUE ("IsVisibile") -> [w254]
          n84 = constructor class="GMapOverlay"("id"=w258) -> (reference out=w253:refnum<k24>)  [unwired: 3 in, 3 out]
          n85 = property class="GMapControl"(reference=w257) -> (reference out=w255:refnum<k24>, "Overlays"=w256:refnum<k24>)  [unwired: 1 in, 1 out]
          n86 = property class="GMapOverlay"(reference=w253, "IsVisibile"=w254) -> (reference out=w252:refnum<k24>)  [unwired: 1 in, 1 out]
          n87 = invoke class="ObservableCollectionThreadSafe`" method="Add"(reference=w256, "item"=w252) -> ()  [unwired: 2 in, 4 out]
        }
        n88 = Bundle By Name(cluster=w249, "dotNetGMap"=w245, "arrOverlayRefs"=w248) -> (w247:T9)
      }
      frame "POINTS -CREATE LIST (Container)" {
        n89 = call "GPS -Points Collection.vi"() -> ("RefPointsColl"=w260:refnum<k24>)  [unwired: 11 in]
        n90 = Bundle By Name(cluster=w259, "RefPointsColl"=w260) -> (w261:T9)
      }
      frame "MARKERS -CREATE LIST" {
      }
      frame "MAP -MARKER Add Or Rmv" {
        w279 = T11 {"arrLatLngActv"=[], "ptKeyorID"=[], "Add"=FALSE}  # PtLatLn+KywrdOrID
        n91 = Unbundle By Name(w278) -> ("dotNetGMap"=w275:refnum<k24>, "arrOverlayRefs"=w270:refnum<k24>[], "RefPointsColl"=w269:refnum<k24>, "arrLatLngActv"=w268:dbl[][], "arrPointKeyWordOrID"=w267:string[])
        n92 = Variant To Data(type=w279, Variant=w280) -> (data=w265:T11)  [unwired: 1 in, 1 out]
        n93 = Bundle By Name(cluster=T12 {"arrOverlayRefs"=[], "RefPointsColl in"=refnum, "arrPointKeyWordOrID"=[], "PtLatLn+KywrdOrID"={"arrLatLngActv"=[], "ptKeyorID"=[], "Add"=FALSE}, "arrLatLngActv"=[]} ("Inputs"), "arrOverlayRefs"=w270, "RefPointsColl in"=w269, "arrLatLngActv"=w268, "arrPointKeyWordOrID"=w267, "PtLatLn+KywrdOrID"=w265) -> (w266:T12)
        n94 = call "GPS -Markers Add to Collection.vi"(".NET Refnum in"=w275, "Inputs"=w266) -> ("RefPointsColl -OUT"=w277:refnum<k24>, "arrPtKyOrId"=w272:string[], "arrLat|LngActv"=w273:dbl[][], "QFNs"=w274:cluster{"FN":T8, "Data":variant}[])  [unwired: 11 in, 3 out]
        n95 = Bundle By Name(cluster=w278, "RefPointsColl"=w277, "arrLatLngActv"=w273, "arrPointKeyWordOrID"=w272) -> (w276:T9)
      }
      frame "DOWNLOAD -Project Addr" {
      }
      frame "MAP -Marker Update" {
        w284 = 0 ("index")
        n96 = Unbundle By Name(w288) -> ("dotNetGMap"=w296:refnum<k24>, "RefPointsColl"=w291:refnum<k24>)  [unwired: 1 out]
        n97 = property class="GMapControl"(reference=w296) -> (reference out=w286:refnum<k24>, "Overlays"=w295:refnum<k24>)  [unwired: 1 in, 1 out]
        n98 = invoke class="List`1[[GMap.NET.PointLatLng, G" method="get_Item"(reference=w291, "index"=w284) -> ("get_Item"=w290:refnum<k24>)  [unwired: 2 in, 3 out]
        n99 = invoke class="ObservableCollectionThreadSafe`" method="get_Item"(reference=w295, "index"=0) -> ("get_Item"=w293:refnum<k24>)  [unwired: 2 in, 3 out]
        n100 = constructor class="GMarkerGoogle"("p"=w290, "type"=T3."orange_dot" ("EnumMarkerTypes")) -> (reference out=w289:refnum<k24>)  [unwired: 3 in, 4 out]
        n101 = property class="GMapOverlay"(reference=w293) -> ("Markers"=w292:refnum<k24>)  [unwired: 1 in, 2 out]
        n102 = invoke class="ObservableCollectionThreadSafe`" method="set_Item"(reference=w292, "index"=w284, "value"=w289) -> ()  [unwired: 2 in, 5 out]
        n103 = Bundle By Name(cluster=w288, "dotNetGMap"=w286) -> (w287:T9)
      }
      frame "MAP -Save" {
        n104 = Unbundle By Name(w300) -> ("dotNetGMap"=w306:refnum<k24>)
        n105 = invoke class="GMapControl" method="ToImage"(reference=w306) -> (reference out=w302:refnum<k24>, "ToImage"=w307:refnum<k24>)  [unwired: 2 in, 1 out]
        n106 = call "File Dialog"("prompt"="Enter Name to Save Map (*.png)", "default name"="MapName.png") -> ("selected path"=w305:path, "cancelled"=w303:bool)  [unwired: 10 in, 2 out]
        n107 = case shown="거짓" w303 {
          tunnel: w307 -> [w312 _]
          tunnel: w305 -> [w311 _]
          tunnel: [w309 w313] -> w301
          tunnel: w302 -> [w309 w313]
          frame False {
            n108 = Path To String(path=w311) -> (string=w310:string)
            "ImgPath" <- w310
            n109 = invoke class="Image" method="Save"(reference=w312, "filename"=w310) -> ()  [unwired: 2 in, 4 out]
          }
          frame True {
          }
        }
        n110 = Bundle By Name(cluster=w300, "dotNetGMap"=w301) -> (w299:T9)
      }
      frame "MAP -Markers Autofit" {
        n111 = Unbundle By Name(w316) -> ("dotNetGMap"=w315:refnum<k24>)
        n112 = invoke class="GMapControl" method="ZoomAndCenterMarkers"(reference=w315, "overlayId"="OL-Markers") -> ()  [unwired: 2 in, 4 out]
      }
      frame "MAP -Addr to Lat + Lng" {
        w344 = 0 ("index (row)")
        n113 = local read "Addr"() -> (w330:string)
        n114 = local read "Prov"() -> (w348:string)
        n115 = local read "City"() -> (w347:string)
        n116 = Bundle By Name(cluster=T13 {"City"="-1", "State"="", "Addr"="", "EID"=""} ("Inputs"), "City"=w347, "State"=w348, "Addr"=w330) -> (w346:T13)
        n117 = Unbundle By Name(w329) -> ("Inputs.Audited"=w323:bool, "Inputs.ctlMode4GPSTool"=w328:T2, "Inputs.Lat"=w327:string, "Inputs.Lng"=w326:string)
        n118 = call "GPS -Get Coordinates from Address.vi"("Inputs"=w346) -> ("Lat|Lng"=w345:string[][])  [unwired: 10 in]
        n119 = Index Array(array=w345, index (row) #1=w344, index (col) #1=w344, index (row) #2=w344, index (col) #2=1 ("disabled index (col)")) -> (element #1=w333:string, element #2=w332:string)
        n120 = Fract/Exp String To Number(string=w333) -> (number=w325:dbl)  [unwired: 3 in, 1 out]
        n121 = Fract/Exp String To Number(string=w332) -> (number=w324:dbl)  [unwired: 3 in, 1 out]
        n122 = call "GPS -Warn Audited Addr.vi"("ctlMode4GPSTool"=w328, "LatPin"=w327, "LngPin"=w326, "AddrLat"=w325, "AddrLng"=w324, "Audited"=w323) -> ("tbCtlGUI"=w320:enum32{"Position", "Pin Drop", "Addr", "Setup"}, "AddrLat -Out"=w319:dbl, "AddrLng -OUT"=w318:dbl, "LatPin"=→"PinDropLatDblClck":dbl, "LngPin"=→"PinDropLngDblClck":dbl)  [unwired: 9 in]
        "AddrLat" <- w319
        "AddrLng" <- w318
        n123 = property on="tbCtlGUI" class="TabCtl (strict)"("Value"=w320) -> ()  [unwired: 2 in, 2 out]
        n124 = Build Array(w319, w318) -> (w338:dbl[])
        n125 = Build Array(w338) -> (w337:dbl[][])
        n126 = Build Array("999950") -> (w336:string[])
        n127 = Bundle By Name(cluster=T11 {"arrLatLngActv"=[], "ptKeyorID"=[], "Add"=FALSE} ("PtLatLn+KywrdOrID"), "arrLatLngActv"=w337, "ptKeyorID"=w336, "Add"=TRUE) -> (w340:T11)
        n128 = Bundle By Name(cluster=cluster{"FN":T8, "Data":variant} {"FN"=enum."MAP -MARKER Add Or Rmv", "Data"=variant} ("element"), "Data"=w340) -> (w339:cluster{"FN":T8, "Data":variant})
        n129 = Build Array(w339) -> (w334:cluster{"FN":T8, "Data":variant}[])
        n130 = disable-structure shown="Disabled" {
          frame Disabled {
            n131 = local read "Prov"() -> ()  [unwired: 1 in]
            n132 = local read "City"() -> ()  [unwired: 1 in]
          }
          frame Enabled {
          }
        }
      }
      frame "MAP -Markers Clear" {
        n133 = Unbundle By Name(w356) -> ("RefPointsColl"=w352:refnum<k24>, "arrOverlayRefs"=w359:refnum<k24>[])
        n134 = Index Array(array=w359) -> (element=w358:refnum<k24>)  [unwired: 1 in]
        n135 = property class="GMapOverlay"(reference=w358) -> ("Markers"=w357:refnum<k24>)  [unwired: 1 in, 2 out]
        n136 = invoke class="ObservableCollectionThreadSafe`" method="Clear"(reference=w357) -> ()  [unwired: 2 in, 3 out]
        n137 = invoke class="List`1[[GMap.NET.PointLatLng, G" method="Clear"(reference=w352) -> (reference out=w351:refnum<k24>)  [unwired: 2 in, 2 out]
        n138 = Bundle By Name(cluster=w356, "RefPointsColl"=w351, "arrPointKeyWordOrID"=string[] [], "arrLatLngActv"=dbl[][] []) -> (w355:T9)
      }
      frame "AUDIT -Use Marker Shown" {
        n139 = Unbundle By Name(w371) -> ("Inputs.Idx"=w367:i32, "arrOverlayRefs"=w372:refnum<k24>[], "Inputs.ctlMode4GPSTool"=w368:T2)
        n140 = Index Array(array=w372) -> (element=w373:refnum<k24>)  [unwired: 1 in]
        n141 = Format Into String(w367) -> (resulting string=w366:string)  [unwired: 3 in, 1 out]
        n142 = property class="GMapOverlay"(reference=w373) -> ("Markers"=w365:refnum<k24>)  [unwired: 1 in, 2 out]
        n143 = property class="ObservableCollectionThreadSafe`"(reference=w365) -> ("Count"=w363:i32)  [unwired: 1 in, 2 out]
        n144 = Equal To 0?(x=w363) -> (x = 0?=w362:bool)
        n145 = Decrement(x=w363) -> (x-1=w364:i32)
        n146 = case shown="참" w362 {
          tunnel: w371 -> [w395 w400]
          tunnel: [w394 w399] -> w370
          tunnel: [w389 w401] -> w369
          tunnel: w368 -> [_ _]
          tunnel: w366 -> [w387 _]
          tunnel: w365 -> [w377 _]
          tunnel: w364 -> [w376 _]
          tunnel: w361 -> [w375 w406]
          tunnel: [w375 w406] -> _
          frame False {
            w378 = i16 7 ("precision (6)")
            n147 = invoke class="ObservableCollectionThreadSafe`" method="get_Item"(reference=w377, "index"=w376) -> ("get_Item"=w397:refnum<k24>)  [unwired: 2 in, 3 out]
            n148 = property class="GMapMarker"(reference=w397) -> ("Position"=w396:refnum<k24>)  [unwired: 1 in, 2 out]
            n149 = local read "Addr"() -> (w386:string)
            n150 = property class="PointLatLng"(reference=w396) -> ("Lat"=w383:dbl, "Lng"=w382:dbl)  [unwired: 1 in, 2 out]
            n151 = local read "City"() -> (w385:string)
            n152 = local read "Prov"() -> (w384:string)
            n153 = Number To Fractional String(number=w382, precision (6)=w378) -> (F-format string=w380:string)  [unwired: 2 in]
            n154 = Format Into String(format string="NOTE:  Will Use\n------\no Address:\n%s\n\no City = %s\no Province or State = %s\no Lat = %f\no Lng =%f\n\n.... Please Confirm this", w386, w385, w384, w383, w382) -> (resulting string=w392:string)  [unwired: 2 in, 1 out]
            n155 = Number To Fractional String(number=w383, precision (6)=w378) -> (F-format string=w381:string)  [unwired: 2 in]
            n156 = Build Array(w387, w386, w385, w384, w381, w380, "1") -> (w374:string[])
            n157 = Bundle By Name(cluster=w395, "Idx|Addr|City|Prov|Lng|Lat|Checked"=w374) -> (w394:T9)
            n158 = Two Button Dialog(message=w392, 1:"-- Wait, I need to Audit Further  --" ("F button name (\"Cancel\")"), 2:"OK" ("T button name (\"OK\")")) -> (T button?=w388:bool)
            n159 = case shown="참" w388 {
              tunnel: [_ cluster{"FN":T8, "Data":variant}[] [{"FN"=enum."exit", "Data"=variant}] ("QFNs")] -> w389
              frame False {
              }
              frame True {
              }
            }
          }
          frame True {
            n160 = Two Button Dialog(message="NOTE:  Will Use\n------\nThere is no Pin Location on Map.\nWould you like to Cancel Audit\n.... Please Confirm this" ("format string"), 1:"-- Wait, I need to Audit Further  --" ("F button name (\"Cancel\")"), 2:"OK" ("T button name (\"OK\")")) -> (T button?=w402:bool)
            n161 = case shown="참" w402 {
              tunnel: [_ cluster{"FN":T8, "Data":variant}[] [{"FN"=enum."exit", "Data"=variant}] ("QFNs")] -> w401
              tunnel: w400 -> [w407 w410]
              tunnel: [w407 w409] -> w399
              frame False {
              }
              frame True {
                n162 = Build Array("-1") -> (w408:string[])
                n163 = global read "GLOBAL -Project MAIN.vi" "EvntAuditAddr"() -> (w413:refnum<user-event>)
                n164 = Generate User Event(user event=w413, event data cluster=w408) -> ()  [unwired: 2 in, 2 out]
                n165 = Bundle By Name(cluster=w410, "Idx|Addr|City|Prov|Lng|Lat|Checked"=w408) -> (w409:T9)
              }
            }
          }
        }
      }
      frame "PIN DROP -Get Nearest" {
        n166 = local read "PinDropLngDblClck"() -> (w418:dbl)
        n167 = local read "PinDropLatDblClck"() -> (w419:dbl)
        n168 = local read "AddrLng"() -> (w416:dbl)
        n169 = local read "AddrLat"() -> (w417:dbl)
        n170 = property on="tbCtlGUI" class="TabCtl (strict)"() -> ("Value"=w421:enum32{"Position", "Pin Drop", "Addr", "Setup"})  [unwired: 2 in, 2 out]
        n171 = Bundle By Name(cluster=T14 {" # Pts"=5, "PinDropLatDblClck"=0.0, "PinDropLngDblClck"=0.0, "AddrLat"=0.0, "AddrLng"=0.0, "tbVw"=enum."Position"} ("Inputs"), "tbVw"=w421, "# Pts"="# Pts", "PinDropLatDblClck"=w419, "PinDropLngDblClck"=w418, "AddrLat"=w417, "AddrLng"=w416) -> (w415:T14)
        n172 = call "GPS -Nearest Points to Lat Lng.vi"("Inputs"=w415, "error in (no error)"=w424) -> ("error out"=w423:errorcluster)  [unwired: 13 in]
      }
      frame "error" {
      }
      frame "exit" {
        n173 = global write "GLBL -GPSLocation.vi" "EXIT-GPS"(TRUE ("EXIT-GPS")) -> ()
      }
    }
    n174 = call "STTM Q MGR -GPS LOCATION.vi"("ERROR"=w55, "Q-IN"=w46, "QFNs"=w48, "Enum"=w47) -> ()  [unwired: 12 in]
  }
  "error out" <- w41
  n175 = global write "GLBL -GPSLocation.vi" "EXIT-GPS"(w40) -> ()
  n176 = while {
    tunnel: w40 -> [_]
    tunnel: w23 -> [w430]
    stop <- w431 stop-if-true
    n177 = event shown="[5] \"btnZoom+Center\": 값 변경" {
      selector: _ -> [_ _ _ _ _ _ _ _ _ _ _ _ _ _]
      dyn-events: _ -> [_ _ _ _ _ _ _ _ _ _ _ _ _ _]
      timeout: _ -> [_ _ _ _ _ _ _ _ _ _ _ _ _ _]
      tunnel: w430 -> [_ _ w433 w441 w443 w445 _ w448 w450 w452 w454 w456 w458 w460]
      event Timeout {
        n178 = event-data() -> ()  [unwired: 1 in, 3 out]
      }
      event "dotNetGMap": Mouse Up {
        n179 = event-data() -> ()  [unwired: 1 in, 1 out]
      }
      event "Refersh": Value Change {
        n180 = event-data() -> ()  [unwired: 1 in, 2 out]
        n181 = Enqueue Element(queue=w433, element=cluster{"FN":T8, "Data":variant} {"FN"=enum."preinit01", "Data"=variant}) -> ()  [unwired: 2 in, 3 out]
      }
      event "PinDropMrkr": Value Change {
        n182 = event-data() -> ()  [unwired: 1 in, 1 out]
        n183 = Format Into String("PinDropMrkr") -> (resulting string=w438:string)  [unwired: 3 in, 1 out]
        n184 = Bundle By Name(cluster=T16 {"r|c"=[], "ID"="", "MrkName"=""} ("Cluster"), "ID"="999950", "MrkName"=w438) -> (w435:T16)
        n185 = Bundle By Name(cluster=cluster{"FN":T8, "Data":variant} {"FN"=enum."MAP -Marker Update", "Data"=variant} ("element"), "Data"=w435) -> (w434:cluster{"FN":T8, "Data":variant})
        n186 = Enqueue Element(queue=w441, element=w434) -> ()  [unwired: 2 in, 3 out]
      }
      event "SaveImage": Value Change {
        n187 = event-data() -> ()  [unwired: 1 in, 1 out]
        n188 = Enqueue Element(queue=w443, element=cluster{"FN":T8, "Data":variant} {"FN"=enum."MAP -Save", "Data"=variant}) -> ()  [unwired: 2 in, 3 out]
      }
      event "btnZoom+Center": Value Change {
        n189 = event-data() -> ()  [unwired: 1 in, 4 out]
        n190 = Enqueue Element(queue=w445, element=cluster{"FN":T8, "Data":variant} {"FN"=enum."MAP -Markers Autofit", "Data"=variant}) -> ()  [unwired: 2 in, 3 out]
      }
      event Mouse Down? {
        n191 = event-data() -> ("Coords"=→"Coords":T5)  [unwired: 1 in]
        n192 = event-data() -> ()  [unwired: 2 in, 1 out]
      }
      event "cmbProviders": Value Change {
        n193 = event-data() -> ()  [unwired: 1 in, 6 out]
        n194 = Enqueue Element(queue=w448, element=cluster{"FN":T8, "Data":variant} {"FN"=enum."SET -Provider", "Data"=variant}) -> ()  [unwired: 2 in, 3 out]
      }
      event "Get Lat+Lng": Value Change {
        n195 = event-data() -> ()  [unwired: 1 in, 6 out]
        n196 = Enqueue Element(queue=w450, element=cluster{"FN":T8, "Data":variant} {"FN"=enum."MAP -Addr to Lat + Lng", "Data"=variant}) -> ()  [unwired: 2 in, 3 out]
      }
      event "GetNearPts": Value Change {
        n197 = event-data() -> ()  [unwired: 1 in, 6 out]
        n198 = Enqueue Element(queue=w452, element=cluster{"FN":T8, "Data":variant} {"FN"=enum."PIN DROP -Get Nearest", "Data"=variant}) -> ()  [unwired: 2 in, 3 out]
      }
      event "ClearMarkers", "GetNearPtsDyn": Value Change {
        n199 = event-data() -> ()  [unwired: 1 in, 6 out]
        n200 = Enqueue Element(queue=w454, element=cluster{"FN":T8, "Data":variant} {"FN"=enum."MAP -Markers Clear", "Data"=variant}) -> ()  [unwired: 2 in, 3 out]
      }
      event "Zoom": Value Change {
        n201 = event-data() -> ()  [unwired: 1 in, 2 out]
        n202 = Enqueue Element(queue=w456, element=cluster{"FN":T8, "Data":variant} {"FN"=enum."SET -SCALE", "Data"=variant}) -> ()  [unwired: 2 in, 3 out]
      }
      event "btnUseMarkerShown": Value Change {
        n203 = event-data() -> ()  [unwired: 1 in, 6 out]
        n204 = Enqueue Element(queue=w458, element=cluster{"FN":T8, "Data":variant} {"FN"=enum."AUDIT -Use Marker Shown", "Data"=variant}) -> ()  [unwired: 2 in, 3 out]
      }
      event "btnCancel": Value Change {
        n205 = event-data() -> ()  [unwired: 1 in, 6 out]
        n206 = flat-sequence {
          tunnel: w460 -> [w463]
          tunnel: [w463] -> w459
          frame #0 {
            n207 = global read "GLOBAL -Project MAIN.vi" "EvntAuditAddr"() -> (w464:refnum<user-event>)
            n208 = Generate User Event(user event=w464, event data cluster=string[] ["-1"] ("event data")) -> ()  [unwired: 2 in, 2 out]
          }
        }
        n209 = Enqueue Element(queue=w459, element=cluster{"FN":T8, "Data":variant} {"FN"=enum."exit", "Data"=variant}) -> ()  [unwired: 2 in, 3 out]
      }
    }
    n210 = global read "GLBL -GPSLocation.vi" "EXIT-GPS"() -> (w431:bool)
  }
  n211 = Unbundle By Name(w39) -> ("dotNetGMap"=w35:refnum<k24>, "VIRef"=w38:refnum<vi>)
  n212 = Release Queue(queue=w31, force destroy? (F)=TRUE) -> ()  [unwired: 1 in, 3 out]
  n213 = invoke class="VI" method="FP.Close"(reference=w38) -> (reference out=w36:refnum<vi>)  [unwired: 2 in, 2 out]
  n214 = Close Reference(reference=w35) -> ()  [unwired: 1 in, 1 out]
  n215 = Close Reference(reference=w36) -> ()  [unwired: 1 in, 1 out]
